vi "Get FP By Reference.vi"(8 "error in (no error)":errorcluster, 11 "VI Refnum":refnum<vi>) -> (0 "error out":errorcluster, 1 "Found":bool, 2 "WFP Name":string, 3 "Web FP Out":refnum<class "Web Front Panel.lvclass">)   [LabVIEW 2017, in "Front Panel Publisher.lvlib" / "Front Panel Manager.lvclass"]
uses:
  Front Panel Manager.lvclass
  Web Front Panel_class/Web Front Panel.lvclass
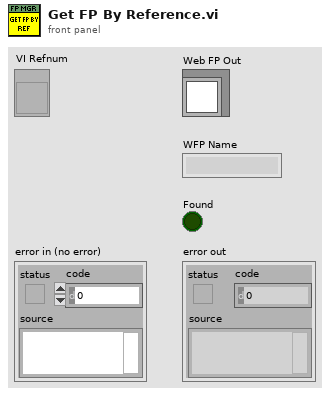
[diagram p1: front panel]
types:
  T1 = typedef "Front Panel Publisher.lvlib/Front Panel Manager.lvclass/Object Attributes.ctl" = cluster{"WebFrontPanels":refnum<class "Web Front Panel.lvclass">[], "WFP Names":string[], "Root folder":path, "Websocket Info":T2}
  T2 = typedef "Front Panel Publisher.lvlib/Front Panel Manager.lvclass/Websocket Info.ctl" = cluster{"Hostname":string, "Port":u16}
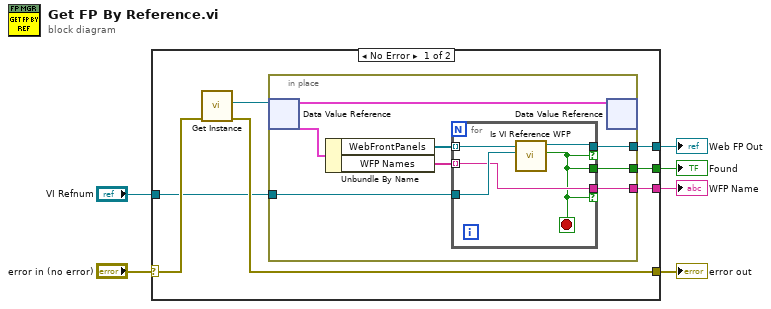
[diagram p0: block diagram]
diagram:
  n1 = case shown="No Error" "error in (no error)" {
    selector: "error in (no error)" -> [w13 w26]
    tunnel: [w12 w26] -> w5
    tunnel: "VI Refnum" -> [w10 _]
    tunnel: [w9 _] -> w4
    tunnel: [w8 _] -> w3
    tunnel: [w7 _] -> w1
    frame No Error {
      n2 = call "Get Instance.vi"("error in (no error)"=w13) -> ("error out"=w12:errorcluster, "DVRRefOut"=w11:refnum<data-value>)  [unwired: 6 in, 3 out]
      n3 = in-place {
        in-place-border: w10 -> [w18]
        in-place-border: [w17] -> w9
        in-place-border: [w16] -> w8
        in-place-border: [w14] -> w7
        n4 = in-place-dvr #1(w11) -> (w20:T1)  [unwired: 1 out]
        n5 = Unbundle By Name(w20) -> ("WebFrontPanels"=w19:refnum<class "Web Front Panel.lvclass">[], "WFP Names"=w15:string[])
        n6 = for {
          tunnel: w19 -> [w25] mode=indexing
          tunnel: w18 -> [w23]
          tunnel: [w24] -> w17 if=w21
          tunnel: [w21] -> w16
          tunnel: w15 -> [w22] mode=indexing
          tunnel: [w22] -> w14 if=w21
          stop <- w21 stop-if-true
          n7 = call "Is VI Reference WFP.vi"("VI Refnum"=w23, "Web FP In"=w25) -> ("VI Reference Is WFP"=w21:bool, "Web FP Out"=w24:refnum<class "Web Front Panel.lvclass">)  [unwired: 7 in, 1 out]
        }
        n8 = in-place-dvr #1(w20) -> ()  [unwired: 2 out]
      }
    }
    frame Error {
    }
  }
  "error out" <- w5
  "Web FP Out" <- w4
  "Found" <- w3
  "WFP Name" <- w1
